vi "Instrument Level Processing.vi"(8 "error in (no error)":errorcluster, 9 "Instrument Level Controls in":T4, 10 "Voice Level Processing in":T2, 11 "MIDI Controls in":T3=variant(dbl 0.0)) -> (0 "error out":errorcluster, 2 "Instrument Level Processing out":T1)   [LabVIEW 2014, in "mySynthesizer.lvlib" / "Instrument Level Processing.lvlib"]
uses:
  Instrument Level Processing.lvlib
  Instrument Level Controls/Instrument Level Controls.ctl
  MIDI Controls/MIDI Controls.ctl
  Voice Level Processing/Voice Level Processing.ctl
  Instrument Level Processing.ctl
  MIDI Controls/MIDI Controls.lvlib
  Instrument Level Controls/Instrument Level Controls.lvlib
  Voice Level Processing/Voice Level Processing.lvlib
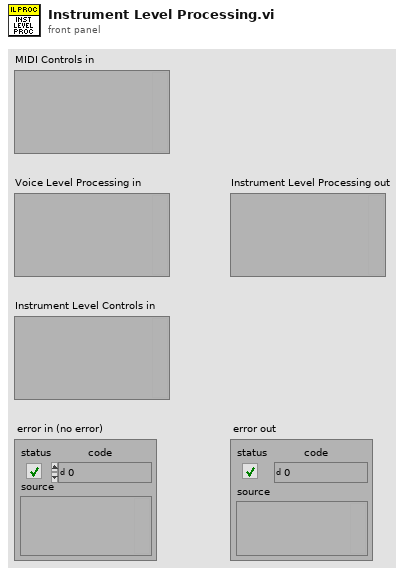
[diagram p1: front panel]
types:
  T1 = typedef "mySynthesizer.lvlib/Instrument Level Processing.lvlib/Instrument Level Processing.ctl" = variant
  T2 = typedef "mySynthesizer.lvlib/Voice Level Processing.lvlib/Voice Level Processing.ctl" = variant
  T3 = typedef "mySynthesizer.lvlib/MIDI Controls.lvlib/MIDI Controls.ctl" = variant
  T4 = typedef "mySynthesizer.lvlib/Instrument Level Controls.lvlib/Instrument Level Controls.ctl" = variant
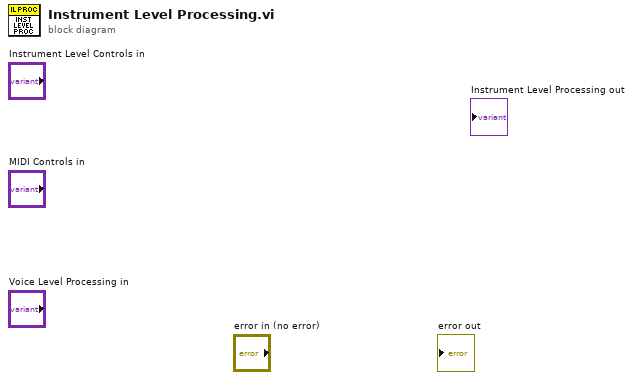
[diagram p0: block diagram]
diagram:
